vi "Select Function.vi"(11 "Numeric":i32) -> (3 "result":i32)   [LabVIEW 2014]
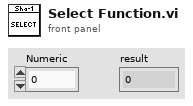
[diagram p1: front panel]
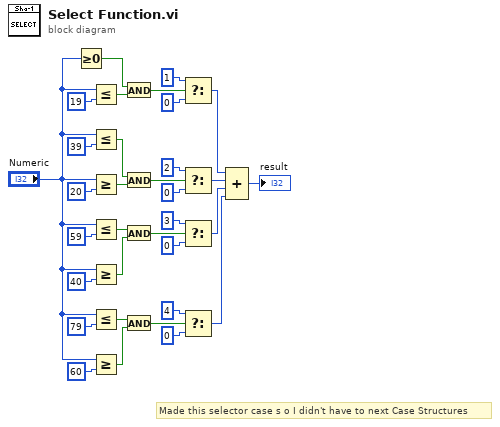
[diagram p0: block diagram]
diagram:
  # "Made this selector case s o I didn't have to next Case Structures"
  n1 = Greater Or Equal To 0?(x="Numeric") -> (x >= 0?=w30:bool)
  n2 = Less Or Equal?(x="Numeric", y=19) -> (x <= y?=w29:bool)
  n3 = Less Or Equal?(x="Numeric", y=39) -> (x <= y?=w25:bool)
  n4 = Greater Or Equal?(x="Numeric", y=20) -> (x >= y?=w26:bool)
  n5 = Less Or Equal?(x="Numeric", y=59) -> (x <= y?=w18:bool)
  n6 = Greater Or Equal?(x="Numeric", y=40) -> (x >= y?=w19:bool)
  n7 = Less Or Equal?(x="Numeric", y=79) -> (x <= y?=w14:bool)
  n8 = Greater Or Equal?(x="Numeric", y=60) -> (x >= y?=w15:bool)
  n9 = And(x=w30, y=w29) -> (x .and. y?=w32:bool)
  n10 = And(x=w25, y=w26) -> (x .and. y?=w23:bool)
  n11 = And(x=w18, y=w19) -> (x .and. y?=w12:bool)
  n12 = And(x=w14, y=w15) -> (x .and. y?=w8:bool)
  n13 = Select(t=1, s=w32, f=0) -> (s? t:f=w5:i32)
  n14 = Select(t=2, s=w23, f=0) -> (s? t:f=w4:i32)
  n15 = Select(t=3, s=w12, f=0) -> (s? t:f=w3:i32)
  n16 = Select(t=4, s=w8, f=0) -> (s? t:f=w2:i32)
  n17 = Compound Arithmetic op=ADD(w5, w4, w3, w2) -> (→"result":i32)
